vi "Handle Error.vi"(8 "error in (no error)":errorcluster, 11 "Simulated Wash Display Console Actor in":refnum<class "Simulated Wash Display Console Actor.lvclass">) -> (0 "error out":errorcluster, 2 "stop actor?":bool=TRUE, 3 "Simulated Wash Display Console Actor out":refnum<class "Simulated Wash Display Console Actor.lvclass">)   [LabVIEW 2019, in "Simulated Wash Display Console Actor.lvlib" / "Simulated Wash Display Console Actor.lvclass"]
doc: "(<B>Filename</B>: Actor Framework.lvlib:Actor.lvclass:Handle Error.vi)\n\nDefines how the actor handles an error that occurred while processing a message. By default, this method does nothing except stop the actor."
uses:
  Simulated Wash Display Console Actor.lvclass
  C:/Program Files (x86)/National Instruments/LabVIEW 2019/vi.lib/ActorFramework/Actor/Actor.lvclass
  Car Wash Controller Actor/Car Wash Controller Actor/Error Levels.ctl
  <vilib>/ActorFramework/Actor/Actor.lvclass/Actor.ctl
  Car Wash Controller Actor/Car Wash Controller Actor Messages/Centrialize Error Handling Msg/Centrialize Error Handling Msg.lvclass/Centrialize Error Handling Msg.ctl
  <vilib>/ActorFramework/Message Enqueuer/Message Enqueuer.lvclass/Message Enqueuer.ctl
  <vilib>/ActorFramework/Message Enqueuer/Enqueue.vi
  Car Wash Controller Actor/Car Wash Controller Actor Messages/Centrialize Error Handling Msg/Centrialize Error Handling Msg.lvclass
  C:/Program Files (x86)/National Instruments/LabVIEW 2019/vi.lib/ActorFramework/Message/Message.lvclass
  <vilib>/ActorFramework/Message Priority Queue/Priority Enqueue.vi
  Abstract Washer Display Console Actor/Abstract Washer Display Console Actor/Washer Display Console Actor.lvclass
  <vilib>/ActorFramework/Actor/Actor.lvclass
  Car Wash Controller Actor/Car Wash Controller Actor/Car Wash Controller Actor.lvclass
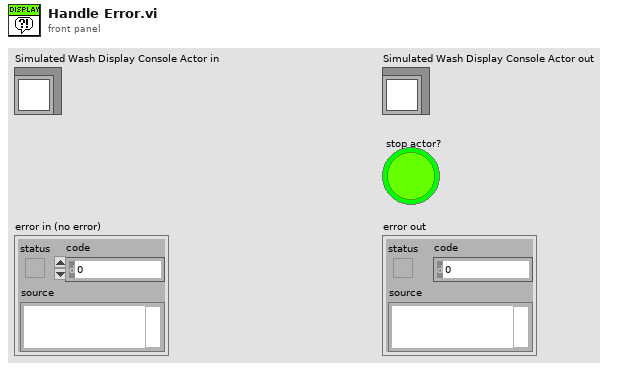
[diagram p1: front panel]
types:
  T1 = typedef "Car Wash Controller Actor.lvlib/Car Wash Controller Actor.lvclass/Error Levels.ctl" = enum16{"Minor Error", "Wash Cycle Error", "System Error"}
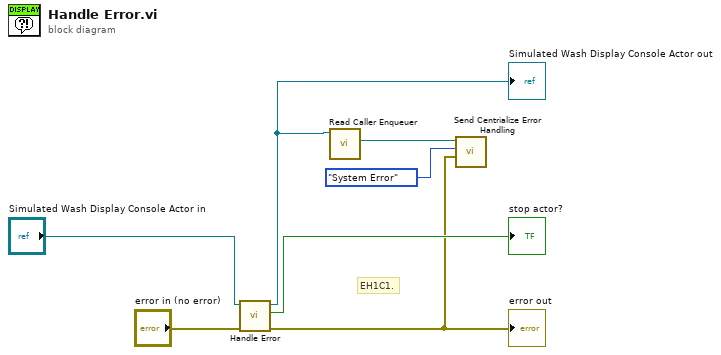
[diagram p0: block diagram]
diagram:
  # "EH1C1."
  n1 = call-parent "Handle Error.vi"("error in (no error)"="error in (no error)", "Actor in"="Simulated Wash Display Console Actor in") -> ("error out"=w1:errorcluster, "stop actor?"=→"stop actor?":bool, "Actor out"=w2:refnum<class "Simulated Wash Display Console Actor.lvclass">)  [unwired: 7 in]
  "Simulated Wash Display Console Actor out" <- w2
  "error out" <- w1
  n2 = call <vilib>:"Read Caller Enqueuer.vi"("Actor"=w2) -> ("Caller Enqueuer"=w4:refnum<class "Message Enqueuer.lvclass">)  [unwired: 10 in]
  n3 = call "Send Centrialize Error Handling.vi"("Error"=w1, "Error Level"=Error_Levels."System Error", "Message Enqueuer"=w4) -> ()  [unwired: 7 in, 2 out]
